vi "Motor_Drehrichtung.vi"(8 "error in":errorcluster, 9 "drehrichtung":u8, 10 "Motorwahl":string(combo)="0", 11 "VISA resource name in":refnum<visa-resource-name>) -> (0 "error out":errorcluster, 2 "Gesendeter Code":string, 3 "VISA resource name out":refnum<visa-resource-name>)   [LabVIEW 2014]
panel:
  in  "Steuercode":string="d"
  in  "Kennung - RN-Motorsteuerung":string="#rm"
  # "0=links\n1=rechts"
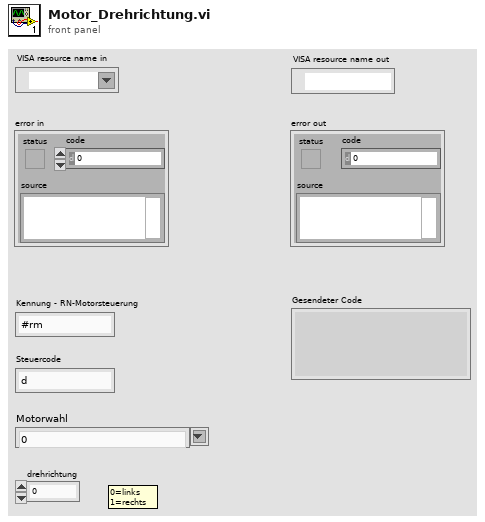
[diagram p1: front panel]
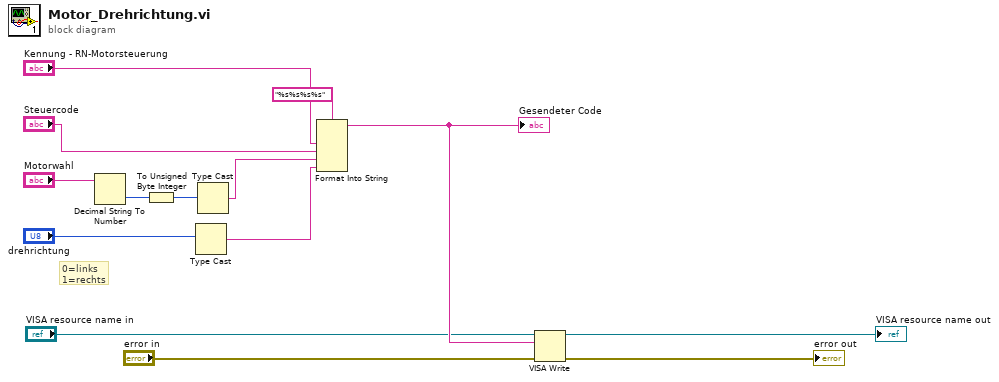
[diagram p0: block diagram]
diagram:
  # "0=links\n1=rechts"
  n1 = Decimal String To Number(string="Motorwahl") -> (number=w13:i32)  [unwired: 2 in, 1 out]
  n2 = To Unsigned Byte Integer(number=w13) -> (unsigned 8bit integer=w12:u8)
  n3 = Type Cast(x="drehrichtung") -> (*(type *) &x=w7:string)  [unwired: 1 in]
  n4 = Type Cast(x=w12) -> (*(type *) &x=w8:string)  [unwired: 1 in]
  n5 = Format Into String(format string="%s%s%s%s", "Kennung - RN-Motorsteuerung", "Steuercode", w8, w7) -> (resulting string=w5:string)  [unwired: 2 in, 1 out]
  "Gesendeter Code" <- w5
  n6 = VISA Write(VISA resource name="VISA resource name in", write buffer=w5, error in (no error)="error in") -> (VISA resource name out=→"VISA resource name out":refnum<visa-resource-name>, error out=→"error out":errorcluster)  [unwired: 1 out]
